vi "Point In Rectangle.vi"(10 "rect":T1, 11 "point":T2) -> (3 "point in rect":bool)   [LabVIEW 2023]
doc: "See if the point is within the rect."
uses:
  <vilib>/Utility/miscctls.llb/LVPoint32TypeDef.ctl
  <vilib>/Utility/miscctls.llb/LVRectTypeDef.ctl
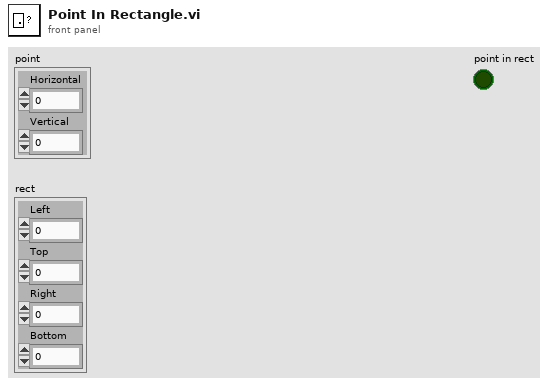
[diagram p1: front panel]
types:
  T1 = typedef "LVRectTypeDef.ctl" = cluster{"Left":i16, "Top":i16, "Right":i16, "Bottom":i16}
  T2 = typedef "LVPoint32TypeDef.ctl" = cluster{"Horizontal":i32, "Vertical":i32}
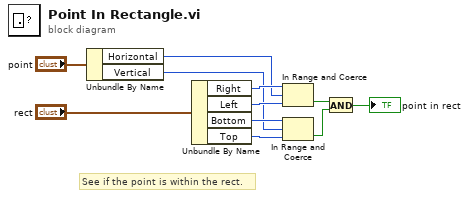
[diagram p0: block diagram]
diagram:
  # "See if the point is within the rect."
  n1 = Unbundle By Name("point") -> ("Horizontal"=w7:i32, "Vertical"=w4:i32)
  n2 = Unbundle By Name("rect") -> ("Right"=w9:i16, "Left"=w8:i16, "Bottom"=w6:i16, "Top"=w5:i16)
  n3 = In Range and Coerce(upper limit=w9, x=w7, lower limit=w8) -> (In Range?=w3:bool)  [unwired: 1 out]
  n4 = In Range and Coerce(upper limit=w6, x=w4, lower limit=w5) -> (In Range?=w2:bool)  [unwired: 1 out]
  n5 = And(x=w3, y=w2) -> (x .and. y?=→"point in rect":bool)
